vi "ModeSelectorfromRecipe.vi"(9 "Pin_Index":dbl, 10 "Vbat_Index":dbl, 11 "Vcc_Index":dbl) -> (0 "Mode":string, 1 "Pin_Index 2":i32, 2 "Vbat_Index 2":i32, 3 "Vcc_Index 2":i32)   [LabVIEW 2014]
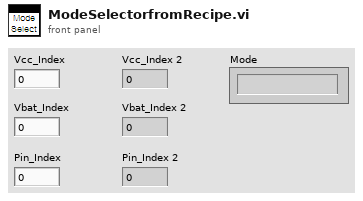
[diagram p1: front panel]
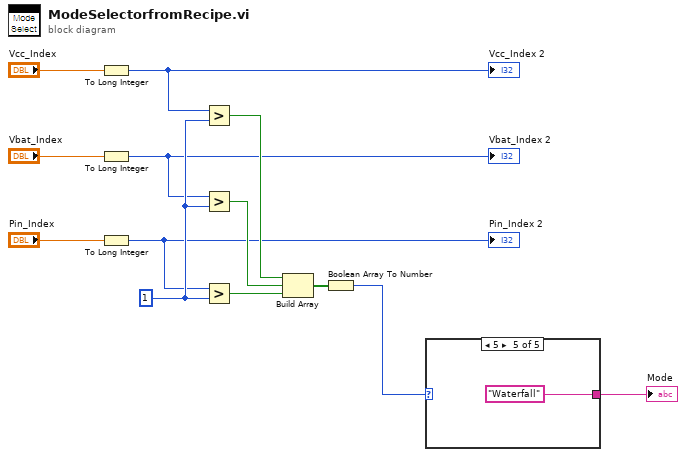
[diagram p0: block diagram]
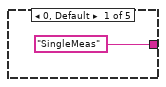
[diagram p2: hidden frame]
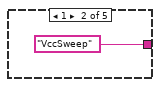
[diagram p3: hidden frame]
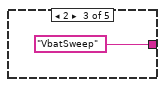
[diagram p4: hidden frame]
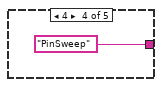
[diagram p5: hidden frame]
diagram:
  w10 = 1 ("y")
  n1 = To Long Integer(number="Vcc_Index") -> (32bit integer=w4:i32)
  "Vcc_Index 2" <- w4
  n2 = To Long Integer(number="Vbat_Index") -> (32bit integer=w5:i32)
  "Vbat_Index 2" <- w5
  n3 = To Long Integer(number="Pin_Index") -> (32bit integer=w6:i32)
  "Pin_Index 2" <- w6
  n4 = Greater?(x=w4, y=w10) -> (0:w7:bool)
  n5 = Greater?(x=w5, y=w10) -> (0:w8:bool)
  n6 = Greater?(x=w6, y=w10) -> (0:w9:bool)
  n7 = Build Array(w7, w8, w9) -> (w3:bool[])
  n8 = Boolean Array To Number(Boolean array=w3) -> (number=w2:u32)
  n9 = case shown="5" w2 {
    tunnel: ["SingleMeas" "VccSweep" "VbatSweep" "PinSweep" "Waterfall"] -> w1
    frame 0, Default {
    }
    frame 1 {
    }
    frame 2 {
    }
    frame 4 {
    }
    frame 5 {
    }
  }
  "Mode" <- w1
